vi "read_回應值_VI.vi"(11 "read buffer":string) -> (3 "回應值":string)   [LabVIEW 2015]
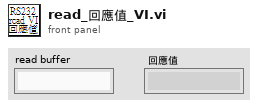
[diagram p1: front panel]
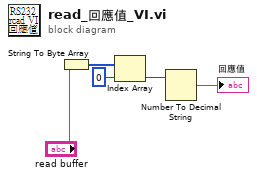
[diagram p0: block diagram]
diagram:
  n1 = String To Byte Array(string="read buffer") -> (unsigned byte array=w4:u8[])
  n2 = Index Array(array=w4, index=0) -> (element=w2:u8)
  n3 = Number To Decimal String(number=w2) -> (decimal integer string=→"回應值":string)  [unwired: 1 in]
